vi "Generate Test Numbers.vi"(0 "Session Handle in":T1, 7 "Test Group":string, 9 "Count to Generate":i32, 11 "error in (no error)":errorcluster) -> (4 "Session Handle out":T1, 8 "Valid Test Numbers":i32[](array[numeric]), 15 "error out":errorcluster)   [LabVIEW 2016]
uses:
  Test Number and Bin Generator.lvclass
  Typedefs/Session Handle.ctl
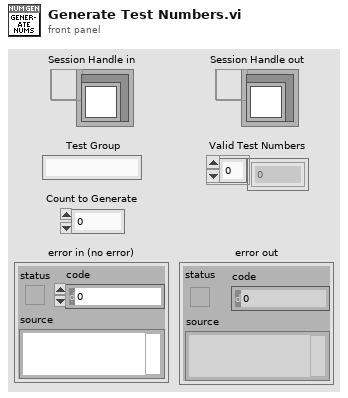
[diagram p1: front panel]
types:
  T1 = typedef "Test Number and Bin Generator.lvclass/Session Handle.ctl" = refnum<data-value>
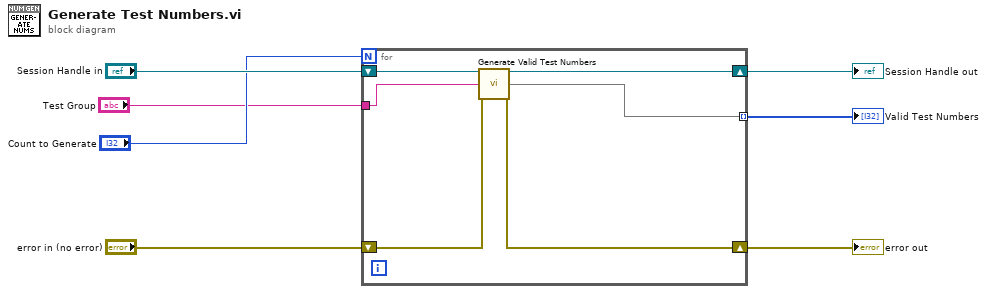
[diagram p0: block diagram]
diagram:
  n1 = for {
    N: "Count to Generate" -> [_]
    shift-right: [w12] -> w5
    shift-left: "error in (no error)" -> [w13]
    shift-right: [w10] -> w4
    shift-left: "Session Handle in" -> [w11]
    tunnel: "Test Group" -> [w9]
    tunnel: [w8] -> w1 mode=indexing
    n2 = call "Generate Valid Test Numbers.vi"("Session Handle in"=w11, "Test Group"=w9, "error in (no error)"=w13) -> ("Session Handle out"=w10:T1, 8:w8, "error out"=w12:errorcluster)  [unwired: 9 in, 1 out]
  }
  "Session Handle out" <- w4
  "error out" <- w5
  "Valid Test Numbers" <- w1
